vi "set_led_half_periods.vi"(8 "error in":errorcluster, 9 "I2C interface":T2, 10 "Half periods (sec)":dbl[](array[numeric]), 11 "Initial phase (degrees)":dbl[](array[numeric])=[0.0, 0.0, 0.0, 0.0, 0.0, 0.0]) -> (0 "error out":errorcluster)   [LabVIEW 2014]
uses:
  i2c_interface.ctl
  fpga_reference.ctl
  Common/fractional_phase.ctl
  i2c_defs.vi
  <vilib>/Utility/error.llb/Error Cluster From Error Code.vi
  <vilib>/rvi/errors/niLvFpgaAdjustHostInterfaceError.vi
  <vilib>/rvi/interface/nirviReadWriteControl/nirviReadWriteControl.xnode
  FPGA Bitfiles/i2cmuxdemux.lvbitx
  NiFpgaLv.dll
panel:
  out "Phase adv":T1[](array[typedef])
  out "Init phase":T1[](array[typedef])
  # "Set half periods (i.e. 1/(2*f)) and initial phase for ASAP LEDs.  Useful for testing and calibration.  Setting to the globals in asap globals.vi restores the defaults."
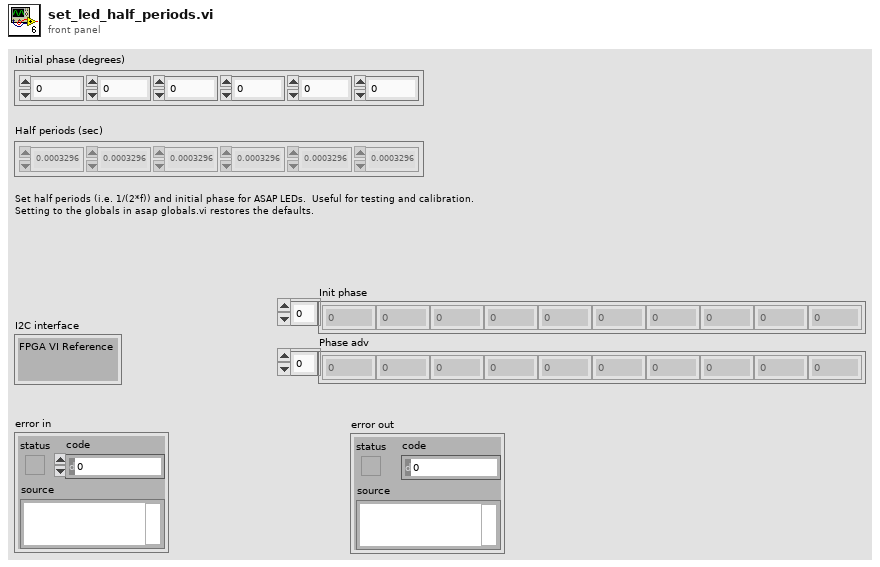
[diagram p1: front panel]
types:
  T1 = typedef "fractional_phase.ctl" = fxp<+,32,1>
  T2 = typedef "i2c_interface.ctl" = cluster{"FPGA VI Reference":T3}
  T3 = typedef "fpga_reference.ctl" = refnum<k20>
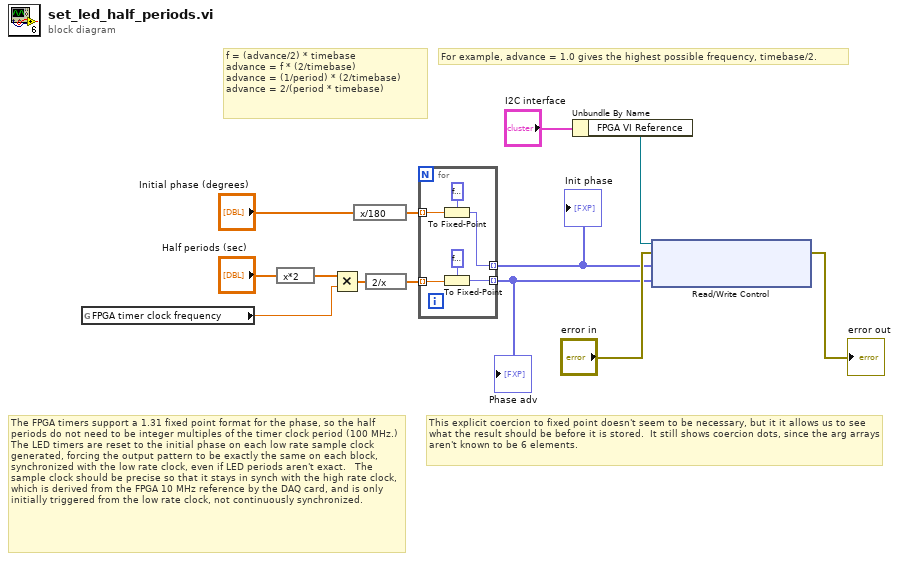
[diagram p0: block diagram]
diagram:
  # "This explicit coercion to fixed point doesn't seem to be necessary, but it it allows us to see what the result should be before it is stored.  It still shows coercion dots, since the arg arrays aren't known to be 6 elements."
  # "For example, advance = 1.0 gives the highest possible frequency, timebase/2."
  # "f = (advance/2) * timebase\nadvance = f * (2/timebase)\nadvance = (1/period) * (2/timebase)\nadvance = 2/(period * timebase)"
  # "The FPGA timers support a 1.31 fixed point format for the phase, so the half periods do not need to be integer multiples of the timer clock period (100 MHz.)  The LED timers are reset to the initial phase on each low rate sample clock generated, forcing the output pattern to be exactly the same on each block, synchronized with the low rate clock, even if LED periods aren't exact.   The sample clock should be precise so that it stays in synch with the high rate clock, which is derived from the FPGA 10 MHz reference by the DAQ card, and is only initially triggered from the low rate clock, not continuously synchronized."
  n1 = global read "i2c_defs.vi" "FPGA timer clock frequency"() -> (w9:dbl)
  n2 = expression code="x*2"("Half periods (sec)") -> (w1:dbl[])
  n3 = Multiply(x=w1, y=w9) -> (x*y=w7:dbl[])
  n4 = expression code="x/180"("Initial phase (degrees)") -> (w5:dbl[])
  n5 = expression code="2/x"(w7) -> (w6:dbl[])
  n6 = for {
    tunnel: w6 -> [w19] mode=indexing
    tunnel: [w18] -> w3 mode=indexing
    tunnel: w5 -> [w17] mode=indexing
    tunnel: [w16] -> w4 mode=indexing
    n7 = To Fixed-Point(fixed-point type=T1 0.0 ("Half period"), number=w17) -> (fixed-point=w16:T1)
    n8 = To Fixed-Point(fixed-point type=T1 0.0 ("Half period"), number=w19) -> (fixed-point=w18:T1)
  }
  "Init phase" <- w4
  "Phase adv" <- w3
  n9 = Unbundle By Name("I2C interface") -> ("FPGA VI Reference"=w12:T3)
  n10 = xnode "Read/Write Control"("FPGA VI Reference In"=w12, "error in"="error in", "ASAP timer initial phase"=w4, "ASAP timer phase advance"=w3) -> ("error out"=→"error out":errorcluster)  [unwired: 1 out]
